vi "frw_edf2array.vi"(10 "block size (3600s)":dbl=3600.0, 11 "file path":path=path "C:/Users/Cassani/Desktop/test_data.edf") -> (1 "2D array":dbl[][](array[numeric]), 2 "fs":dbl, 3 "channel names out":string[](array[string]))   [LabVIEW 2013]
doc: "Reads EDF file and put the data in a 2D array"
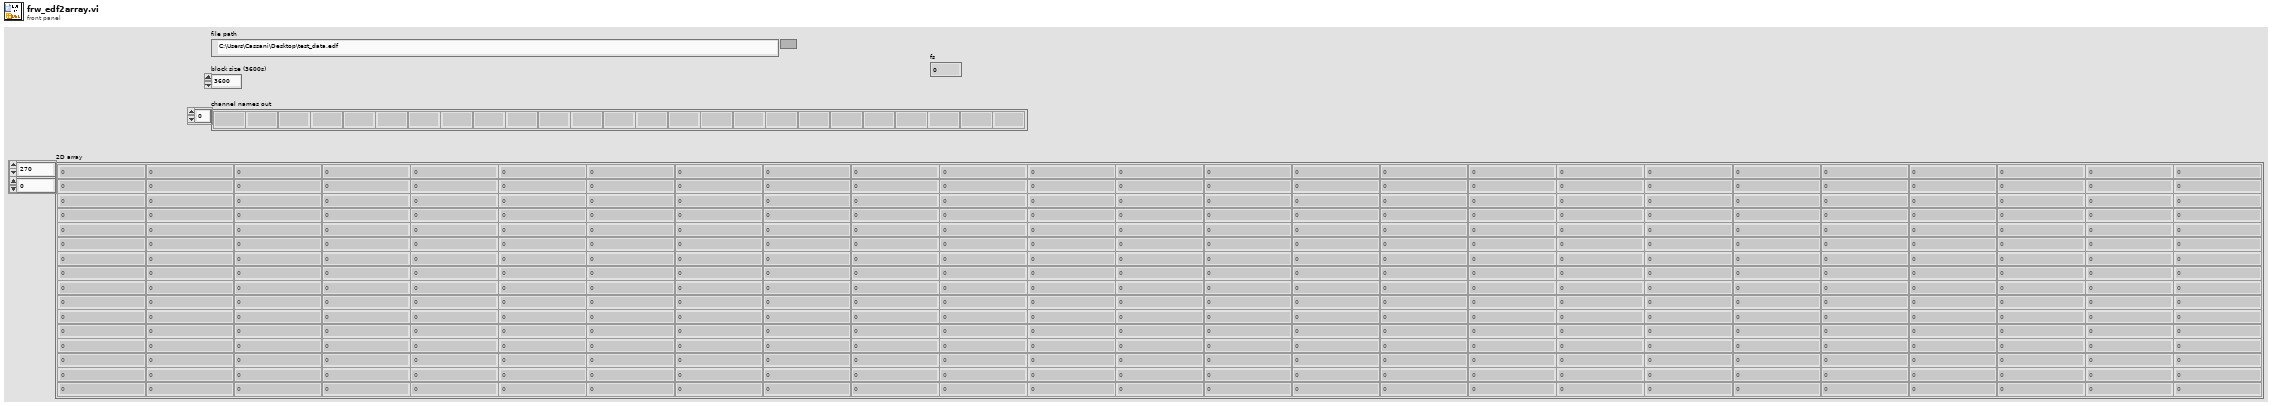
[diagram p1: front panel]
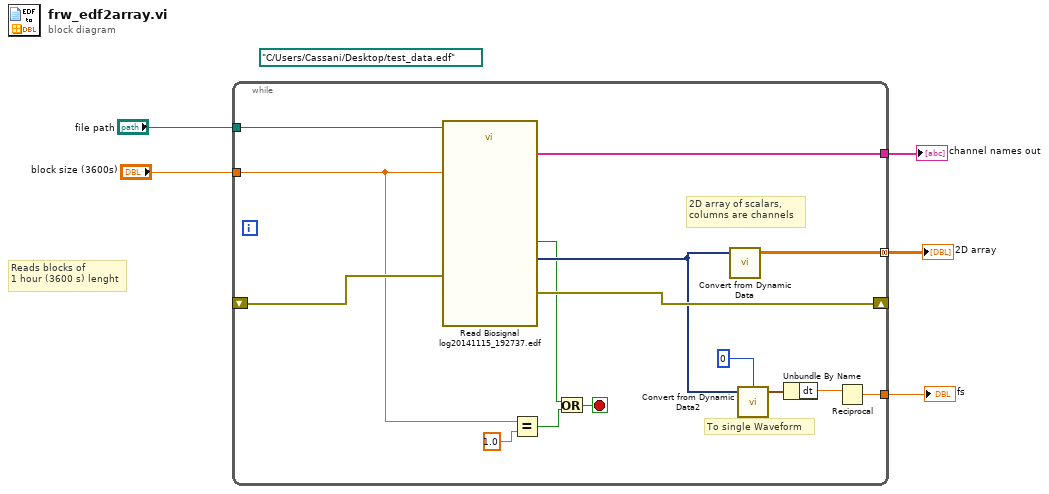
[diagram p0: block diagram]
diagram:
  (unwired) path "C:/Users/Cassani/Desktop/test_data.edf" ("file path")
  # "Reads blocks of\n1 hour (3600 s) lenght"
  n1 = while {
    tunnel: [w20] -> w5 mode=concatenating
    tunnel: [w19] -> w3
    tunnel: "file path" -> [w18]
    shift-right: [w16] -> _
    shift-left: _ -> [w17]
    tunnel: [w12] -> w2
    tunnel: "block size (3600s)" -> [w7]
    stop <- w10 stop-if-true
    # "To single Waveform"
    # "2D array of scalars, \ncolumns are channels"
    n2 = call "Read Biosignal\nlog20141115_192737.edf"("file path"=w18, "error in (no error)"=w17, "block size"=w7) -> ("biosignals"=w15:dynamicdata, "channel names out"=w19:string[], "EOF?"=w9:bool, "error out"=w16:errorcluster)  [unwired: 8 in, 1 out]
    n3 = Equal?(x=w7, y=1.0 ("block size (3600s)")) -> (x = y?=w8:bool)
    n4 = Or(x=w9, y=w8) -> (x .or. y?=w10:bool)
    n5 = call "Convert from Dynamic Data"("Dynamic Data Type"=w15) -> ("Array"=w20:dbl[][])  [unwired: 3 in]
    n6 = call "Convert from Dynamic Data2"("Dynamic Data Type"=w15, "Channel"=0) -> ("Waveform"=w14:waveform(dbl))  [unwired: 2 in]
    n7 = Unbundle By Name(w14) -> ("dt"=w13:dbl)
    n8 = Reciprocal(x=w13) -> (1/x=w12:dbl)
  }
  "2D array" <- w5
  "channel names out" <- w3
  "fs" <- w2
